vi "repair string.vi"(2 "String N":i32[](array[numeric]), 3 "Input String":string[](array[string])) -> (0 "Output String":string[](array[string]), 1 "after item 2":string[](array[string])=["Now dura.", "to dura.", "Repair cost", ""])   [LabVIEW 2016]
panel:
  out "before item":string[](array[string])=["Run time & STEP", "Earn GST", "Energy", "Distance(km)", "Date time", "Shoe Type & Lv.", "Shoe #", "durability", "Δdura"]
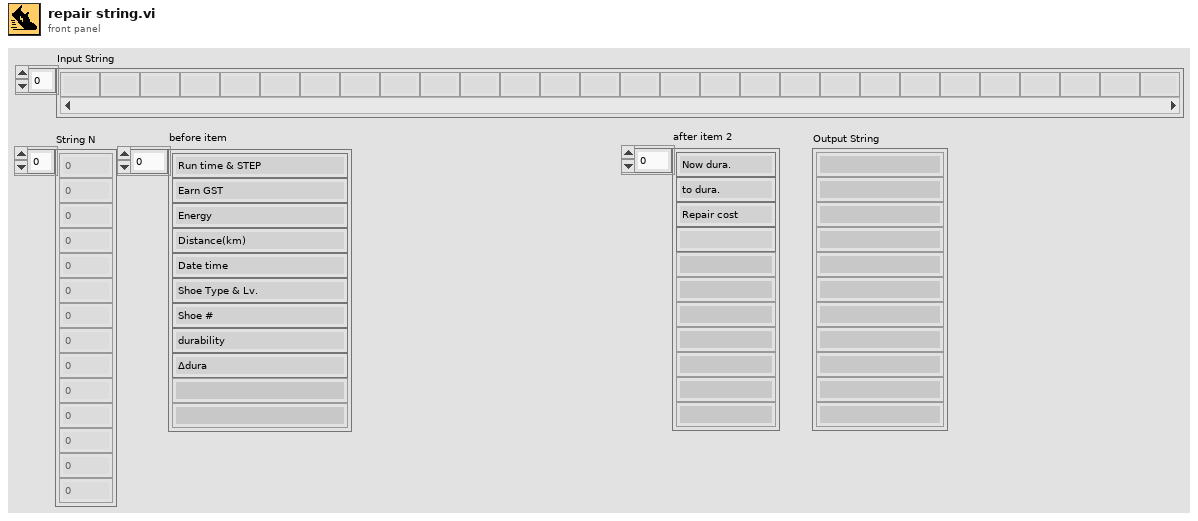
[diagram p1: front panel]
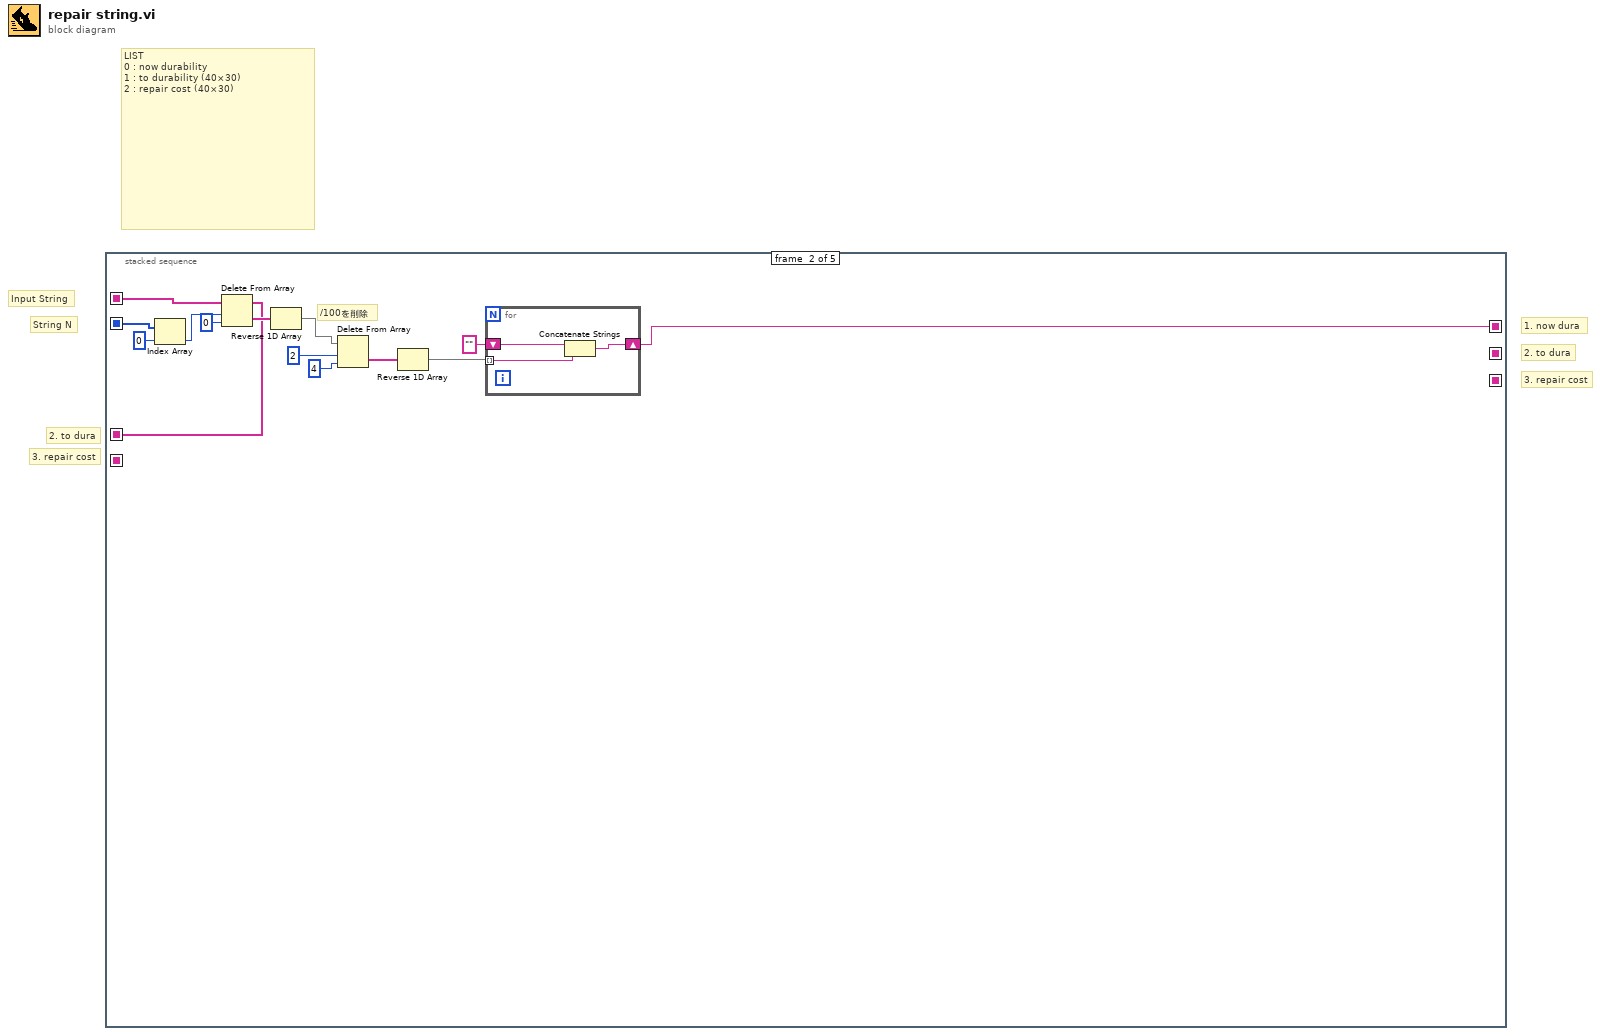
[diagram p0: block diagram]
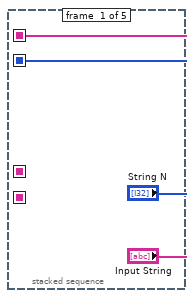
[diagram p2: hidden frame]
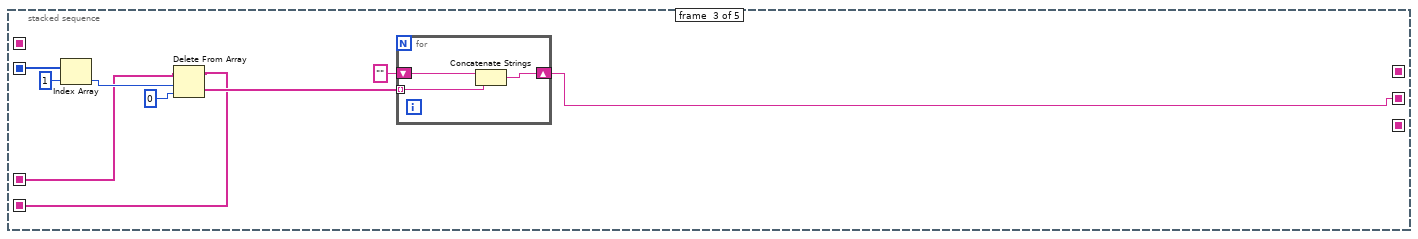
[diagram p3: hidden frame]
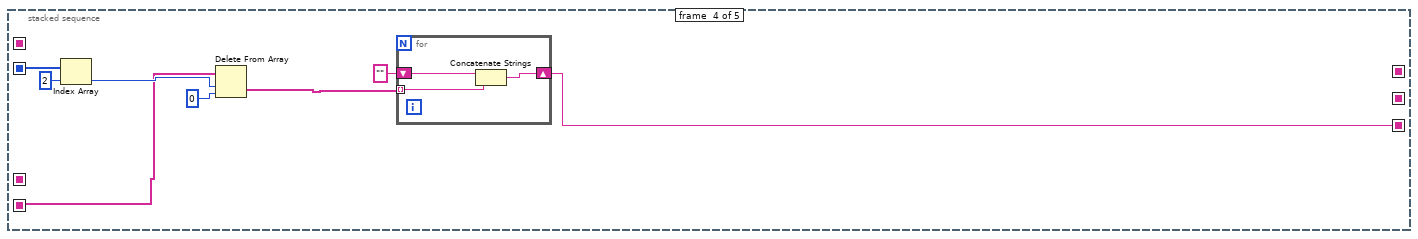
[diagram p4: hidden frame]
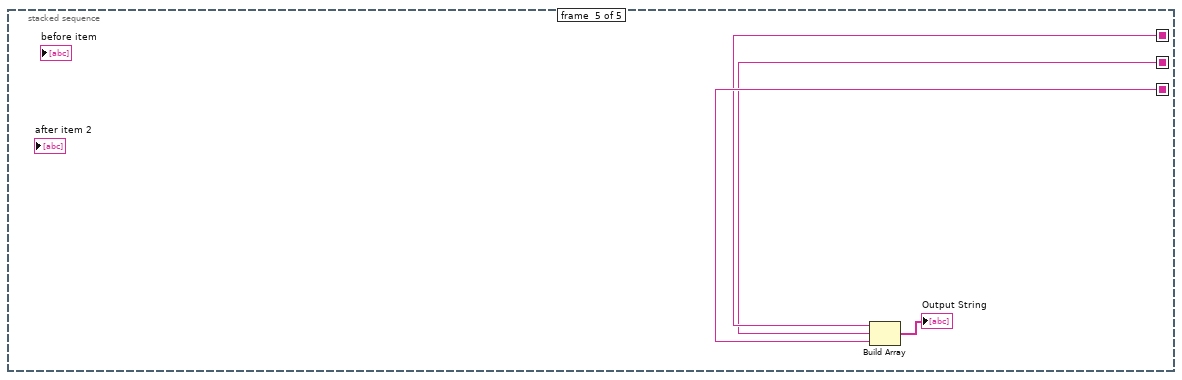
[diagram p5: hidden frame]
diagram:
  # "3. repair cost"
  # "2. to dura"
  # "3. repair cost"
  # "2. to dura"
  # "1. now dura"
  # "LIST\n0 : now durability\n1 : to durability (40×30)\n2 : repair cost (40×30)"
  # "String N"
  # "Input String"
  n1 = stacked-sequence {
    seq-local: ["Input String" _ _ _ _] -> [_ w14 _ _ _]
    seq-local: ["String N" _ _ _ _] -> [_ w12 w24 w36 _]
    seq-local: [_ w3 _ _ _] -> [_ _ w21 _ _]
    seq-local: [_ w15 _ _ _] -> [_ _ _ _ w44]
    seq-local: [_ _ w23 _ _] -> [_ _ _ _ w43]
    seq-local: [_ _ _ w35 _] -> [_ _ _ _ w45]
    seq-local: [_ _ w20 _ _] -> [_ _ _ w32 _]
    frame #0 {
    }
    frame #1 {
      # "/100を削除"
      n2 = Index Array(array=w12, index=0 ("指標")) -> (element=w11:i32)
      n3 = Delete From Array(array=w14, length=w11, index=0) -> (deleted portion=w4:string[], array with subset deleted=w3:string[])
      n4 = Reverse 1D Array(array=w4) -> (reversed array=w8:string[])
      n5 = Delete From Array(array=w8, length=2 ("長さ"), index=4 ("指標")) -> (deleted portion=w7:string[])  [unwired: 1 out]
      n6 = Reverse 1D Array(array=w7) -> (reversed array=w6:string[])
      n7 = for {
        tunnel: w6 -> [w17] mode=indexing
        shift-right: [w19] -> w15
        shift-left: "" -> [w18]
        n8 = Concatenate Strings(w18, w17) -> (w19:string)
      }
    }
    frame #2 {
      n9 = Index Array(array=w24, index=1 ("指標")) -> (element=w22:i32)
      n10 = Delete From Array(array=w21, length=w22, index=0 ("指標")) -> (deleted portion=w25:string[], array with subset deleted=w20:string[])
      n11 = for {
        tunnel: w25 -> [w29] mode=indexing
        shift-right: [w31] -> w23
        shift-left: "" -> [w30]
        n12 = Concatenate Strings(w30, w29) -> (w31:string)
      }
    }
    frame #3 {
      n13 = Index Array(array=w36, index=2 ("指標")) -> (element=w34:i32)
      n14 = Delete From Array(array=w32, length=w34, index=0 ("指標")) -> (deleted portion=w33:string[])  [unwired: 1 out]
      n15 = for {
        tunnel: w33 -> [w40] mode=indexing
        shift-right: [w42] -> w35
        shift-left: "" -> [w41]
        n16 = Concatenate Strings(w41, w40) -> (w42:string)
      }
    }
    frame #4 {
      n17 = Build Array(w44, w43, w45) -> (→"Output String":string[])
    }
  }
